vi "Create Title For CSV.vi"(8 "error in (no error)":errorcluster caption="错误输入（无错误）", 10 "file path":path, 11 "从板数":i32) -> (0 "error out":errorcluster caption="错误输出")   [LabVIEW 2013]
uses:
  <vilib>/Utility/file.llb/Write To Spreadsheet File (string).vi
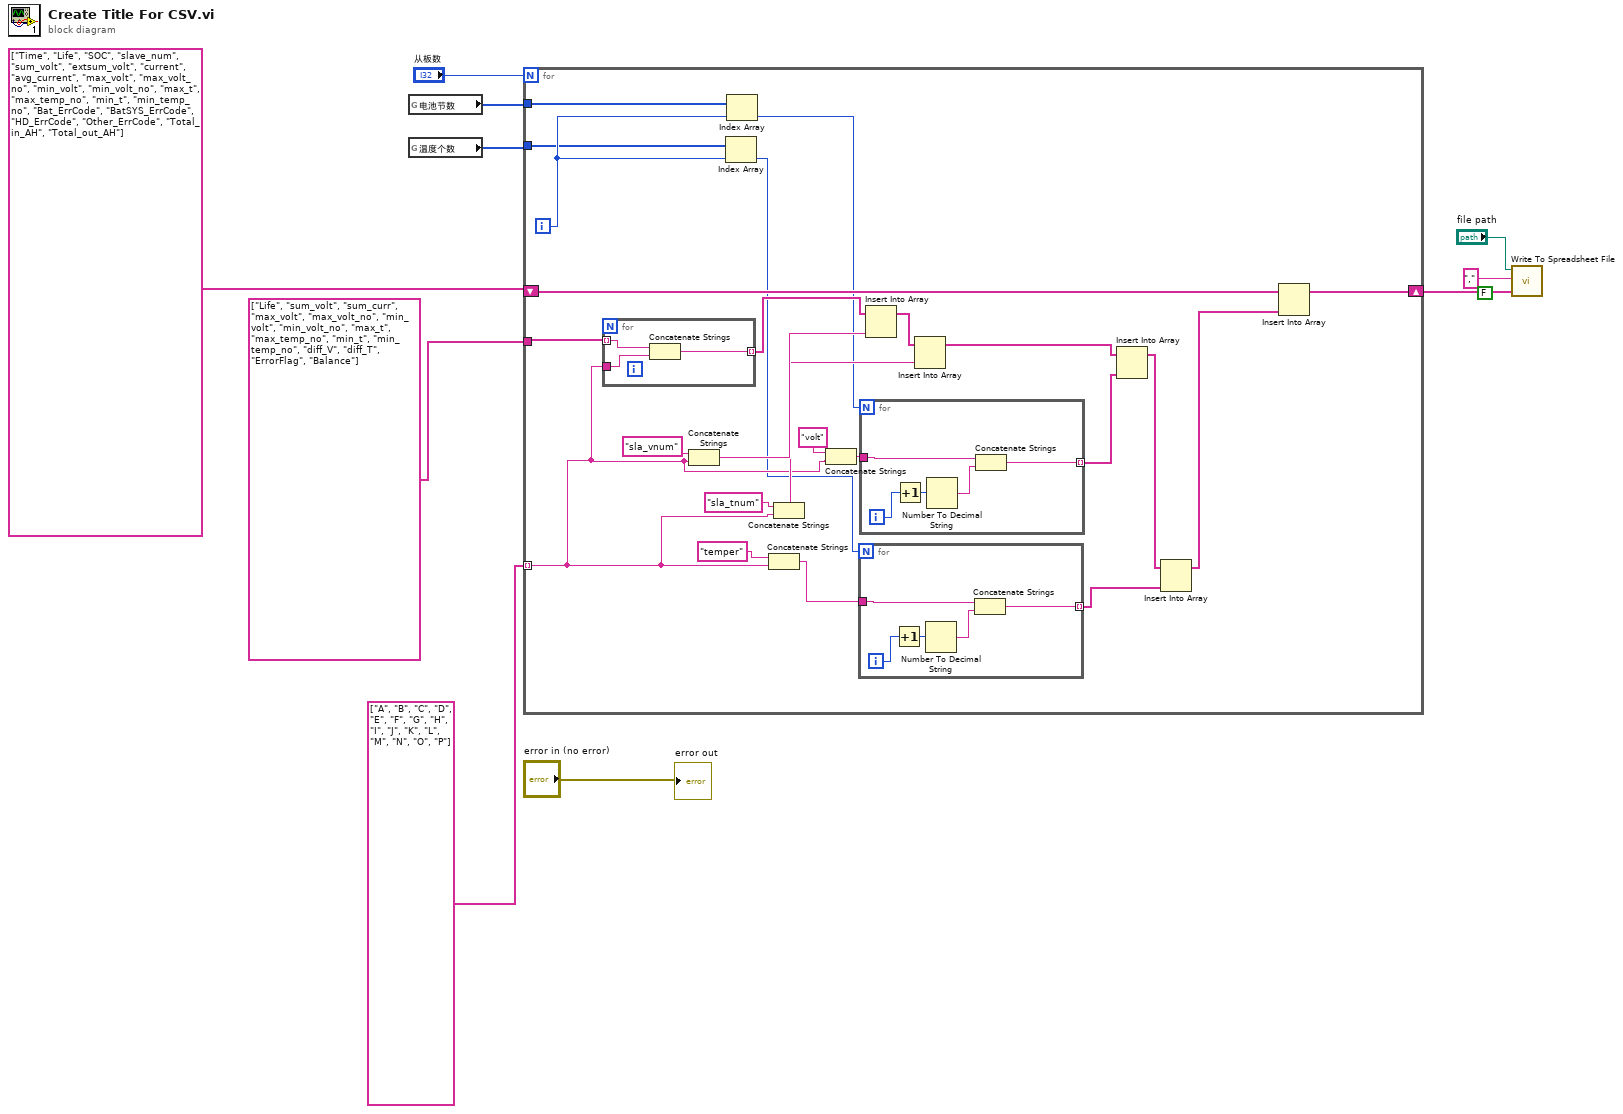
[diagram p0: block diagram]
diagram:
  n1 = global read "从板全局变量.vi" "电池节数"() -> (w3:u8[])
  n2 = global read "从板全局变量.vi" "温度个数"() -> (w2:u8[])
  n3 = for {
    N: "从板数" -> [_]
    tunnel: string[] ["A", "B", "C", "D", "E", "F", "G", "H", "I", "J", "K", "L", "M", "N", "O", "P"] -> [w17] mode=indexing
    tunnel: string[] ["Life", "sum_volt", "sum_curr", "max_volt", "max_volt_no", "min_volt", "min_volt_no", "max_t", "max_temp_no", "min_t", "min_temp_no", "diff_V", "diff_T", "ErrorFlag", "Balance"] -> [w32]
    shift-right: [w20] -> w8
    shift-left: string[] ["Time", "Life", "SOC", "slave_num", "sum_volt", "extsum_volt", "current", "avg_current", "max_volt", "max_volt_no", "min_volt", "min_volt_no", "max_t", "max_temp_no", "min_t", "min_temp_no", "Bat_ErrCode", "BatSYS_ErrCode", "HD_ErrCode", "Other_ErrCode", "Total_in_AH", "Total_out_AH"] -> [w22]
    tunnel: w3 -> [w14]
    tunnel: w2 -> [w12]
    i -> [w16]
    n4 = for {
      tunnel: w32 -> [w48] mode=indexing
      tunnel: w17 -> [w47]
      tunnel: [w46] -> w23 mode=indexing
      n5 = Concatenate Strings(w48, w47) -> (w46:string)
    }
    n6 = Concatenate Strings("sla_vnum" ("字符串"), w17) -> (w31:string)
    n7 = Index Array(array=w12, index=w16) -> (element=w13:u8)
    n8 = Index Array(array=w14, index=w16) -> (element=w15:u8)
    n9 = Concatenate Strings("temper" ("字符串"), w17) -> (w33:string)
    n10 = Concatenate Strings("sla_tnum" ("字符串"), w17) -> (w28:string)
    n11 = Concatenate Strings("volt", w17) -> (w18:string)
    n12 = for {
      N: w13 -> [_]
      tunnel: w33 -> [w38]
      tunnel: [w36] -> w24 mode=indexing
      i -> [w39]
      n13 = Increment(x=w39) -> (x+1=w40:i32)
      n14 = Number To Decimal String(number=w40) -> (decimal integer string=w37:string)  [unwired: 1 in]
      n15 = Concatenate Strings(w38, w37) -> (w36:string)
    }
    n16 = for {
      N: w15 -> [_]
      tunnel: w18 -> [w43]
      tunnel: [w41] -> w26 mode=indexing
      i -> [w44]
      n17 = Increment(x=w44) -> (x+1=w45:i32)
      n18 = Number To Decimal String(number=w45) -> (decimal integer string=w42:string)  [unwired: 1 in]
      n19 = Concatenate Strings(w43, w42) -> (w41:string)
    }
    n20 = Insert Into Array(array=w23, new element=w31) -> (w30:string[])  [unwired: 1 in]
    n21 = Insert Into Array(array=w30, new element=w28) -> (w27:string[])  [unwired: 1 in]
    n22 = Insert Into Array(array=w27, new element=w26) -> (w25:string[])  [unwired: 1 in]
    n23 = Insert Into Array(array=w25, new element=w24) -> (w21:string[])  [unwired: 1 in]
    n24 = Insert Into Array(array=w22, new element=w21) -> (w20:string[])  [unwired: 1 in]
  }
  n25 = call-poly <vilib>:"Write To Spreadsheet File.vi"("delimiter (\\t)"="," ("delimiter (\\t)"), "append to file? (new file:F)"=FALSE, "1D data"=w8, "file path (dialog if empty)"="file path") -> ()  [unwired: 4 in, 1 out]
  "error out" <- "error in (no error)"
